vi "Index Group.vi"(4 "Write?":bool, 8 "error in (no error)":errorcluster, 10 "Group":string, 11 "bt_Blackboard in":refnum<class "bt_Blackboard.lvclass">) -> (0 "error out":errorcluster, 2 "Index":i32, 3 "bt_Blackboard out":refnum<class "bt_Blackboard.lvclass">)   [LabVIEW 2021, in "BT.lvlib" / "bt_Blackboard.lvclass"]
uses:
  bt_Blackboard.lvclass
  bt_Blackboard.lvclass/bt_Blackboard.ctl
  Status Type.ctl
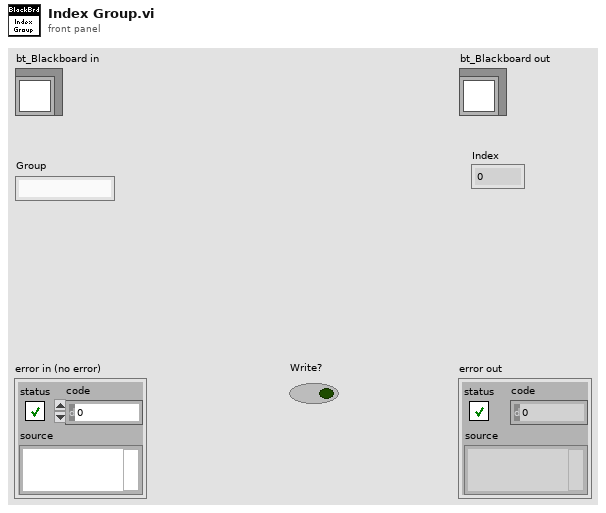
[diagram p1: front panel]
types:
  T1 = typedef "BT.lvlib/bt_Blackboard.lvclass/Status Type.ctl" = cluster{"Read?":bool, "Write?":bool}
  T2 = typedef "BT.lvlib/bt_Blackboard.lvclass/Data DVR Type.ctl" = cluster{"Boolean":cluster{"Tags":refnum<data-value>, "Boolean":refnum<data-value>, "Status":refnum<data-value>}, "String":cluster{"Tags":refnum<data-value>, "String":refnum<data-value>, "Status":refnum<data-value>}, "DBL":cluster{"Tags":refnum<data-value>, "DBL":refnum<data-value>, "Status":refnum<data-value>}, "SGL":cluster{"Tags":refnum<data-value>, "SGL":refnum<data-value>, "Status":refnum<data-value>}, "EXT":cluster{"Tags":refnum<data-value>, "EXT":refnum<data-value>, "Status":refnum<data-value>}, "U8":cluster{"Tags":refnum<data-value>, "U8":refnum<data-value>, "Status":refnum<data-value>}, "U16":cluster{"Tags":refnum<data-value>, "U16":refnum<data-value>, "Status":refnum<data-value>}, "U32":cluster{"Tags":refnum<data-value>, "U32":refnum<data-value>, "Status":refnum<data-value>}, "U64":cluster{"Tags":refnum<data-value>, "U64":refnum<data-value>, "Status":refnum<data-value>}, "I8":cluster{"Tags":refnum<data-value>, "I8":refnum<data-value>, "Status":refnum<data-value>}, "I16":cluster{"Tags":refnum<data-value>, "I16":refnum<data-value>, "Status":refnum<data-value>}, "I32":cluster{"Tags":refnum<data-value>, "I32":refnum<data-value>, "Status":refnum<data-value>}, "I64":cluster{"Tags":refnum<data-value>, "I64":refnum<data-value>, "Status":refnum<data-value>}, "CDBL":cluster{"Tags":refnum<data-value>, "CDBL":refnum<data-value>, "Status":refnum<data-value>}, "CSGL":cluster{"Tags":refnum<data-value>, "CSGL":refnum<data-value>, "Status":refnum<data-value>}, "CEXT":cluster{"Tags":refnum<data-value>, "CEXT":refnum<data-value>, "Status":refnum<data-value>}, "Time":cluster{"Tags":refnum<data-value>, "Time":refnum<data-value>, "Status":refnum<data-value>}, "Variant":cluster{"Tags":refnum<data-value>, "Variant":refnum<data-value>, "Status":refnum<data-value>}, "Waveform":cluster{"Tags":refnum<data-value>, "Waveform":refnum<data-value>, "Status":refnum<data-value>}}
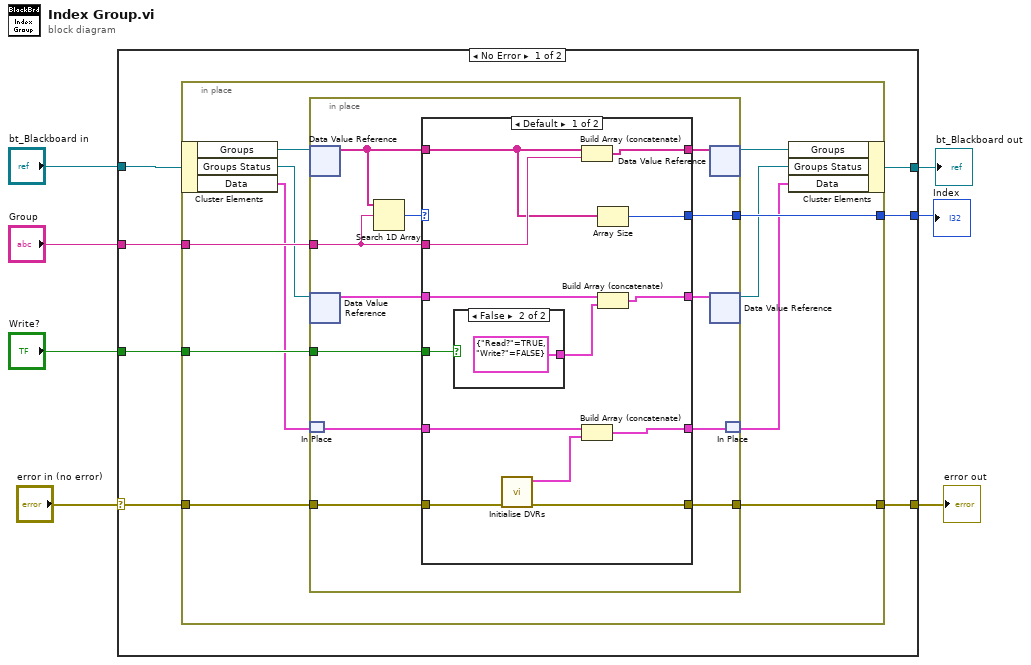
[diagram p0: block diagram]
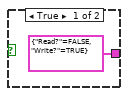
[diagram p2: hidden frame]
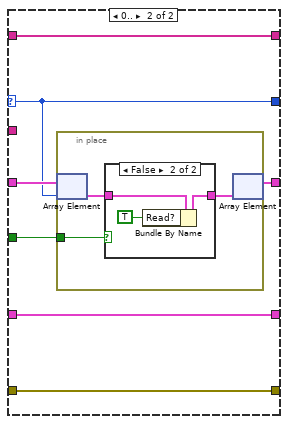
[diagram p3: hidden frame]
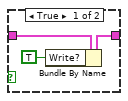
[diagram p4: hidden frame]
diagram:
  n1 = case shown="No Error" "error in (no error)" {
    selector: "error in (no error)" -> [w9 w70]
    tunnel: [w8 w70] -> w6
    tunnel: [w12 w69] -> w4
    tunnel: "bt_Blackboard in" -> [w14 w69]
    tunnel: "Group" -> [w13 _]
    tunnel: [w11 _] -> w2
    tunnel: "Write?" -> [w10 _]
    frame No Error {
      n2 = in-place {
        in-place-border: w13 -> [w23]
        in-place-border: [w22] -> w11
        in-place-border: w10 -> [w20]
        in-place-border: w9 -> [w16]
        in-place-border: [w15] -> w8
        n3 = in-place-cluster #1(w14) -> ("Groups"=w25:refnum<data-value>, "Groups Status"=w21:refnum<data-value>, "Data"=w18:T2[])
        n4 = in-place {
          in-place-border: w23 -> [w33]
          in-place-border: [w34] -> w22
          in-place-border: w20 -> [w30]
          in-place-border: w16 -> [w27]
          in-place-border: [w26] -> w15
          n5 = in-place-dvr #2(w25) -> (w36:string[])  [unwired: 1 out]
          n6 = in-place-dvr #3(w21) -> (w32:T1[])  [unwired: 1 out]
          n7 = in-place-match #4(w18) -> (w29:T2[])
          n8 = Search 1D Array(1D array=w36, element=w33) -> (index of element=w37:i32)  [unwired: 1 in]
          n9 = case shown="Default" w37 {
            selector: w37 -> [_ w57]
            tunnel: w36 -> [w47 w59]
            tunnel: w33 -> [w50 _]
            tunnel: [w49 w59] -> w35
            tunnel: [w48 w57] -> w34
            tunnel: w32 -> [w46 w58]
            tunnel: [w45 w56] -> w31
            tunnel: w30 -> [w43 w55]
            tunnel: w29 -> [w42 w54]
            tunnel: [w41 w54] -> w28
            tunnel: w27 -> [w40 w53]
            tunnel: [w38 w53] -> w26
            frame Default {
              n10 = case shown="False" w43 {
                tunnel: [T1 {"Read?"=FALSE, "Write?"=TRUE} ("Status") T1 {"Read?"=TRUE, "Write?"=FALSE} ("Status")] -> w44
                frame True {
                }
                frame False {
                }
              }
              n11 = call "Initialise DVRs.vi"("error in (no error)"=w40) -> ("error out"=w38:errorcluster, "Data"=w39:T2)  [unwired: 9 in]
              n12 = Build Array (concatenate)(w47, w50) -> (w49:string[])
              n13 = Build Array (concatenate)(w42, w39) -> (w41:T2[])
              n14 = Array Size(array=w47) -> (size(s)=w48:i32)
              n15 = Build Array (concatenate)(w46, w44) -> (w45:T1[])
            }
            frame 0.. {
              n16 = in-place {
                in-place-border: w55 -> [w62]
                n17 = in-place-array #5(w58, w57) -> (w61:T1)
                n18 = case shown="False" w62 {
                  tunnel: w61 -> [w65 w68]
                  tunnel: [w64 w67] -> w60
                  frame True {
                    n19 = Bundle By Name(cluster=w65, "Write?"=TRUE) -> (w64:T1)
                  }
                  frame False {
                    n20 = Bundle By Name(cluster=w68, "Read?"=TRUE ("Write?")) -> (w67:T1)
                  }
                }
                n21 = in-place-array #5(w60) -> (w56:T1[])  [unwired: 1 out]
              }
            }
          }
          n22 = in-place-dvr #2(w35) -> (w24:refnum<data-value>)  [unwired: 1 out]
          n23 = in-place-dvr #3(w31) -> (w19:refnum<data-value>)  [unwired: 1 out]
          n24 = in-place-match #4(w28) -> (w17:T2[])
        }
        n25 = in-place-cluster #1("Groups"=w24, "Groups Status"=w19, "Data"=w17) -> (w12:refnum<class "bt_Blackboard.lvclass">)
      }
    }
    frame Error {
    }
  }
  "error out" <- w6
  "bt_Blackboard out" <- w4
  "Index" <- w2
